vi "SO2 43i Serial Data Recording & DECADEv3.6.vi"() -> ()   [LabVIEW 2014]
uses:
  <vilib>/Instr/_visa.llb/VISA Set IO Buffer Mask.ctl
  <vilib>/Platform/TimedLoop/XDataNode/timing_clust.ctl
  <vilib>/Platform/TimedLoop/XDataNode/nitl_modes.ctl
  <vilib>/Platform/TimedLoop/XDataNode/wakeup.ctl
  C:/Program Files (x86)/National Instruments/LabVIEW 2014/examples/Data Communication/Network Streams/Simple Network Streams/support/Network Stream Command.ctl
  <vilib>/Utility/error.llb/whitespace.ctl
  <vilib>/Instr/_visa.llb/VISA Configure Serial Port (Instr).vi
  <vilib>/Utility/tcp.llb/UDP Multicast Write-Only Open.vi
  <vilib>/platform/TimedLoop/XDataNode/XDataNode.xnode
  <vilib>/Platform/TimedLoop/XDataNode/XDNodeRunTimeDep.lvlib
panel:
  out "Default file name":string
  out "Stop File Write":bool
  out "error out 4":errorcluster
  out "V6":bool
  out "V8":bool
  out "V9":bool
  out "error out 2":errorcluster
  in  "MFC_2 SLPM set value":dbl
  out "Value Read 2":string
  out "status 2":bool
  out "MFC 2":dbl[](array[numeric])
  in  "VISA resource name 3":refnum<visa-resource-name>="ASRL4::INSTR"
  in  "timeout (10sec) 3":u32=3000
  out "error out 3":errorcluster
  in  "MFC_3 SLPM set value":dbl=2.0
  out "Value Read 3":string
  out "status":bool
  out "MFC 3":dbl[](array[numeric])
  in  "VISA resource name 2":refnum<visa-resource-name>="ASRL5::INSTR"
  in  "timeout (10sec) 2":u32=3000
  out "Data Array UDP":string[](array[string])
  out "Slope":dbl=1.0
  out "Offset":dbl
  out "Simulate TWA Conc":dbl
  out "8hr_TWA_limit":i32=490
  out "10mins_STEL_limit":i32=700
  out "Simulate STEL Conc":dbl
  out "Simulate\nconc":bool
  out "q_size 2":i32
  out "8hr_so2_avg 2":dbl=1.0
  out "10min_so2_avg":dbl=1.0
  out "q_size":i32
  in  "Clear Display\nErrors":bool
  in  "dummy2":string="0"
  out "Data Processing":bool
  out "Serial Visa Error":errorcluster
  out "SEPTIC TCP Error Out":errorcluster
  out "TCP packet\nSend to SEPTIC":bool
  out "UDP Time Stamp Offset":i32=1
  out "Data Array TCP":string[](array[string])
  out "UDP packet \nstatus":bool
  out "UDP_Out_Error":errorcluster
  out "FISH TCP Error Out":errorcluster
  out "TCP packet\nSend to FISH":bool
  out "TCP Binary Packet":string
  out "Scan from String Error Counter\nfrom process loop":i32
  out "Read Error Counter\nfrom process loop":i32
  in  "milliseconds to wait":u32=330
  in  "ID":string="µ"
  in  "VISA resource name":refnum<visa-resource-name>="ASRL6::INSTR"
  out "Data In Array":string[](array[string])
  out "UDP_ASCII_Out":string
  out "UDP_Pack_num":u32
  out "Flight Number":string
  in  "dummy1":string="00"
  out "Data String":string
  out "Internal packet":string[](array[string])
  out "RAW DATA":string
  in  "stop":bool
  out "Time taken history":u32(graph)
  out "Max Acq Time diff":u32
  out "Acq Time":u32
  out "Number of Send & Read Error\nfrom Acquire Loop":i32
  out "Command In":string
  # "SO2_conc"
  # "PMT_Volt"
  # "Lamp_Volt"
  # "Lamp_Intensity_Hz"
  # "Internal_Temp_degC"
  # "Reaction_Chamber_Temp_degC"
  # "Reaction_Chamber_Press_mmHg"
  # "Sample_Flow_litre_per_minute"
  # "Flag"
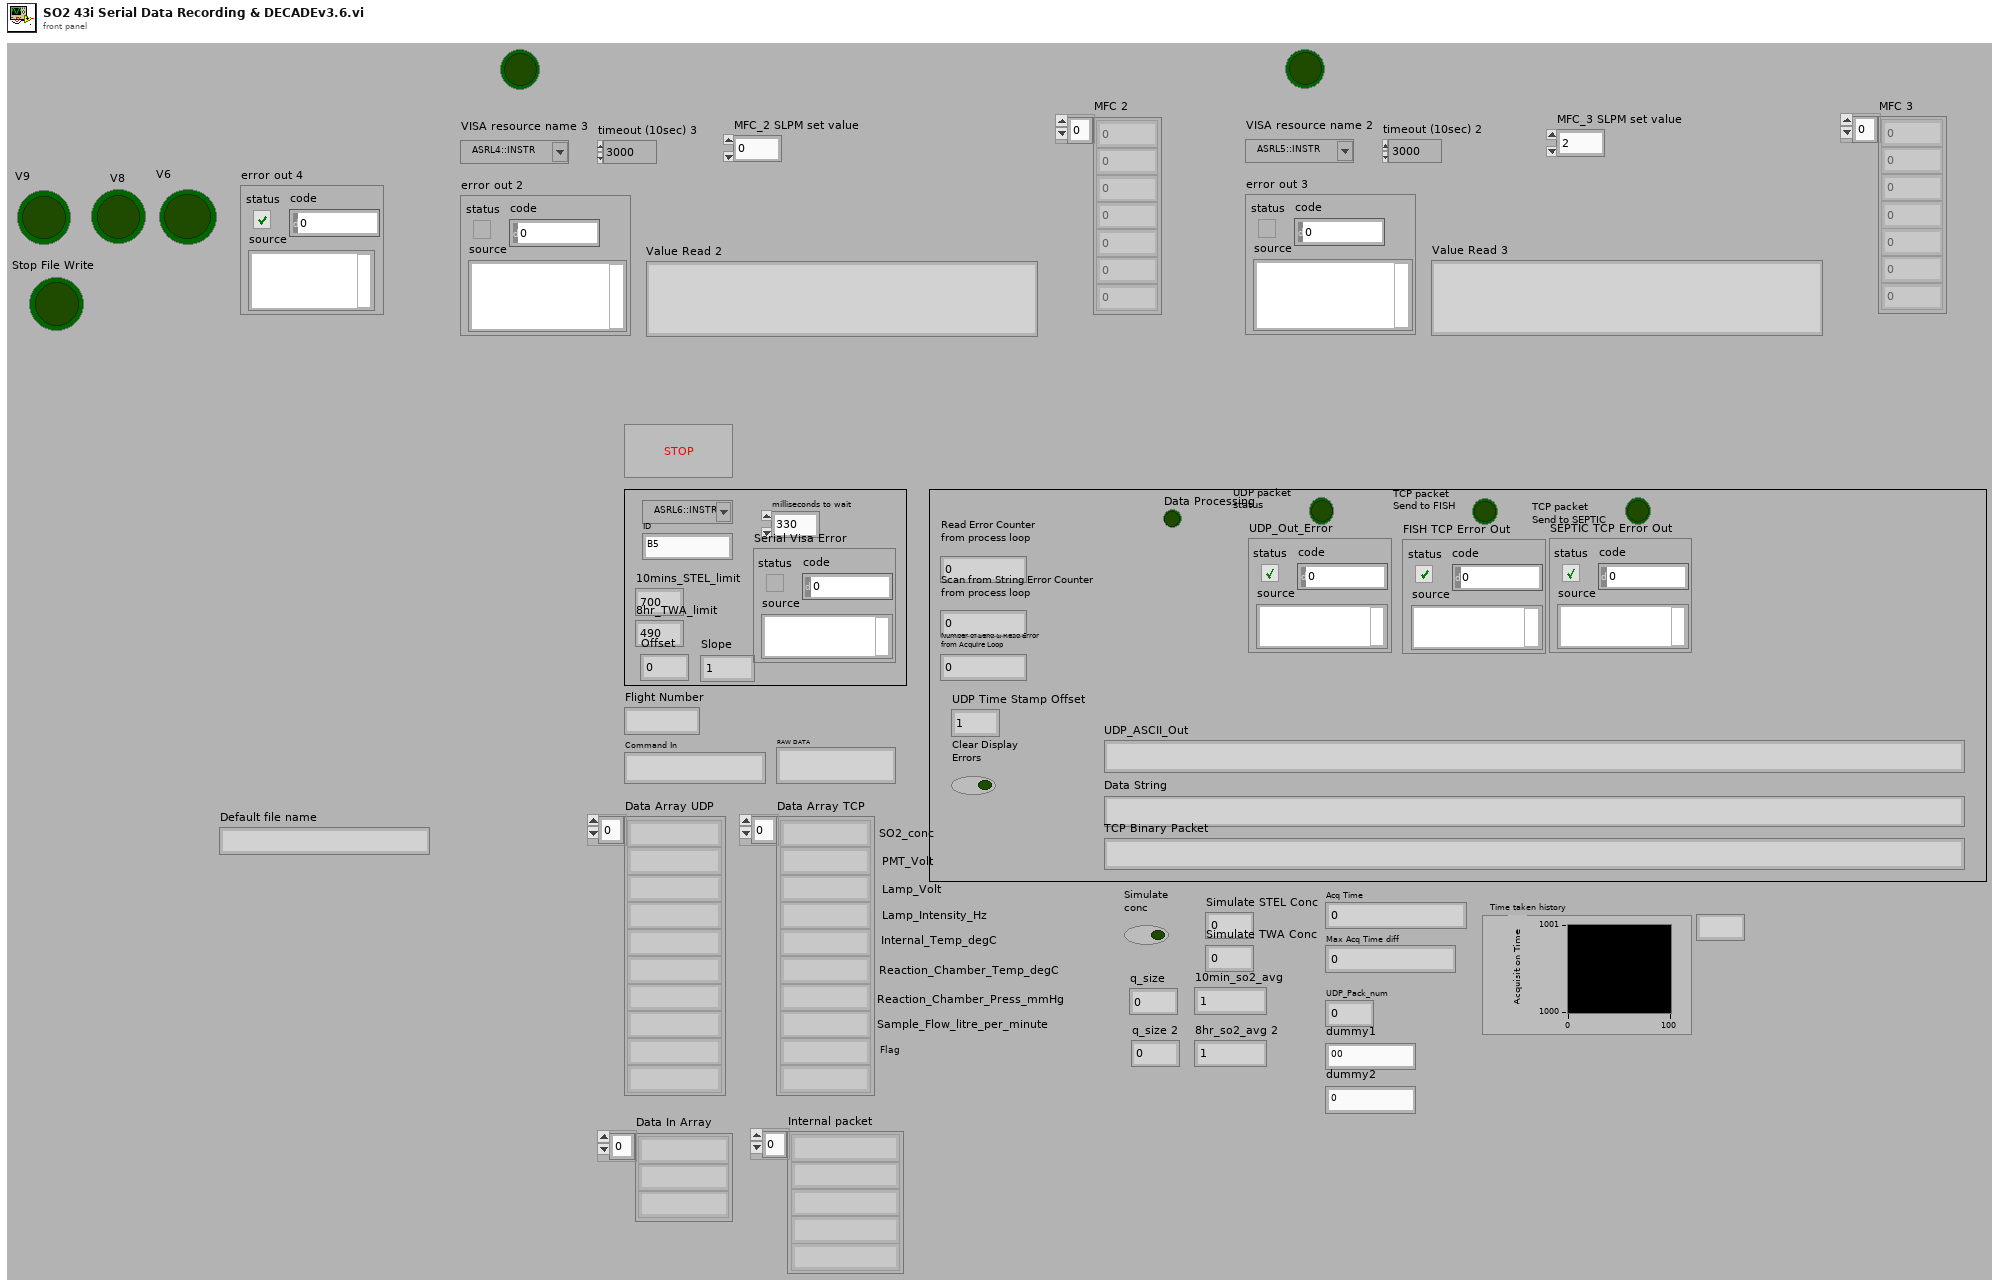
[diagram p1: front panel]
types:
  T1 = typedef "VISA Set IO Buffer Mask.ctl" = u16
  T2 = typedef "Network Stream Command.ctl" = cluster{"Message":string, "Message Data":variant}
  T3 = typedef "XDNodeRunTimeDep.lvlib/timing_clust.ctl" = cluster{"Expected End [f-1]":u64, "Actual End [f-1]":u64, "Finished Late? [f-1]":bool, "Expected End [i-1]":u64, "Actual End [i-1]":u64, "Finished Late? [i-1]":bool, "Expected Start [i]":u64, "Actual Start [i]":u64, "Expected Start [f]":u64, "Actual Start [f]":u64, "Source Name":string, "Structure Name":string, "Period":i64, "Deadline":i64, "Offset":i64, "Start":i64, "Priority":i32, "Timeout":i32, "Mode":T4, "Wakeup Reason":T5, "Error":errorcluster, "Source Type":string, "Secondary Source Type":string, "Global End Time":u64, "Global Start Time":u64, "Frame Duration":u64, "Iteration Duration":u64, "Assigned CPU":i32, "I/O Scan Engine Mode":u32}
  T4 = typedef "XDNodeRunTimeDep.lvlib/nitl_modes.ctl" = enum32{"No Change", "Process missed periods, maintain original phase", "Discard missed periods, maintain original phase", "Process missed periods, ignore original phase", "Discard missed periods, ignore original phase"}
  T5 = typedef "XDNodeRunTimeDep.lvlib/wakeup.ctl" = enum32{"Normal", "Aborted", "Asynchronous wakeup", "Timing source error", "Timed loop error", "Timeout"}
  T6 = enum16{"open", "replace", "create", "open or create", "replace or create", "replace or create with confirmation"}
  T7 = typedef "whitespace.ctl" = u16
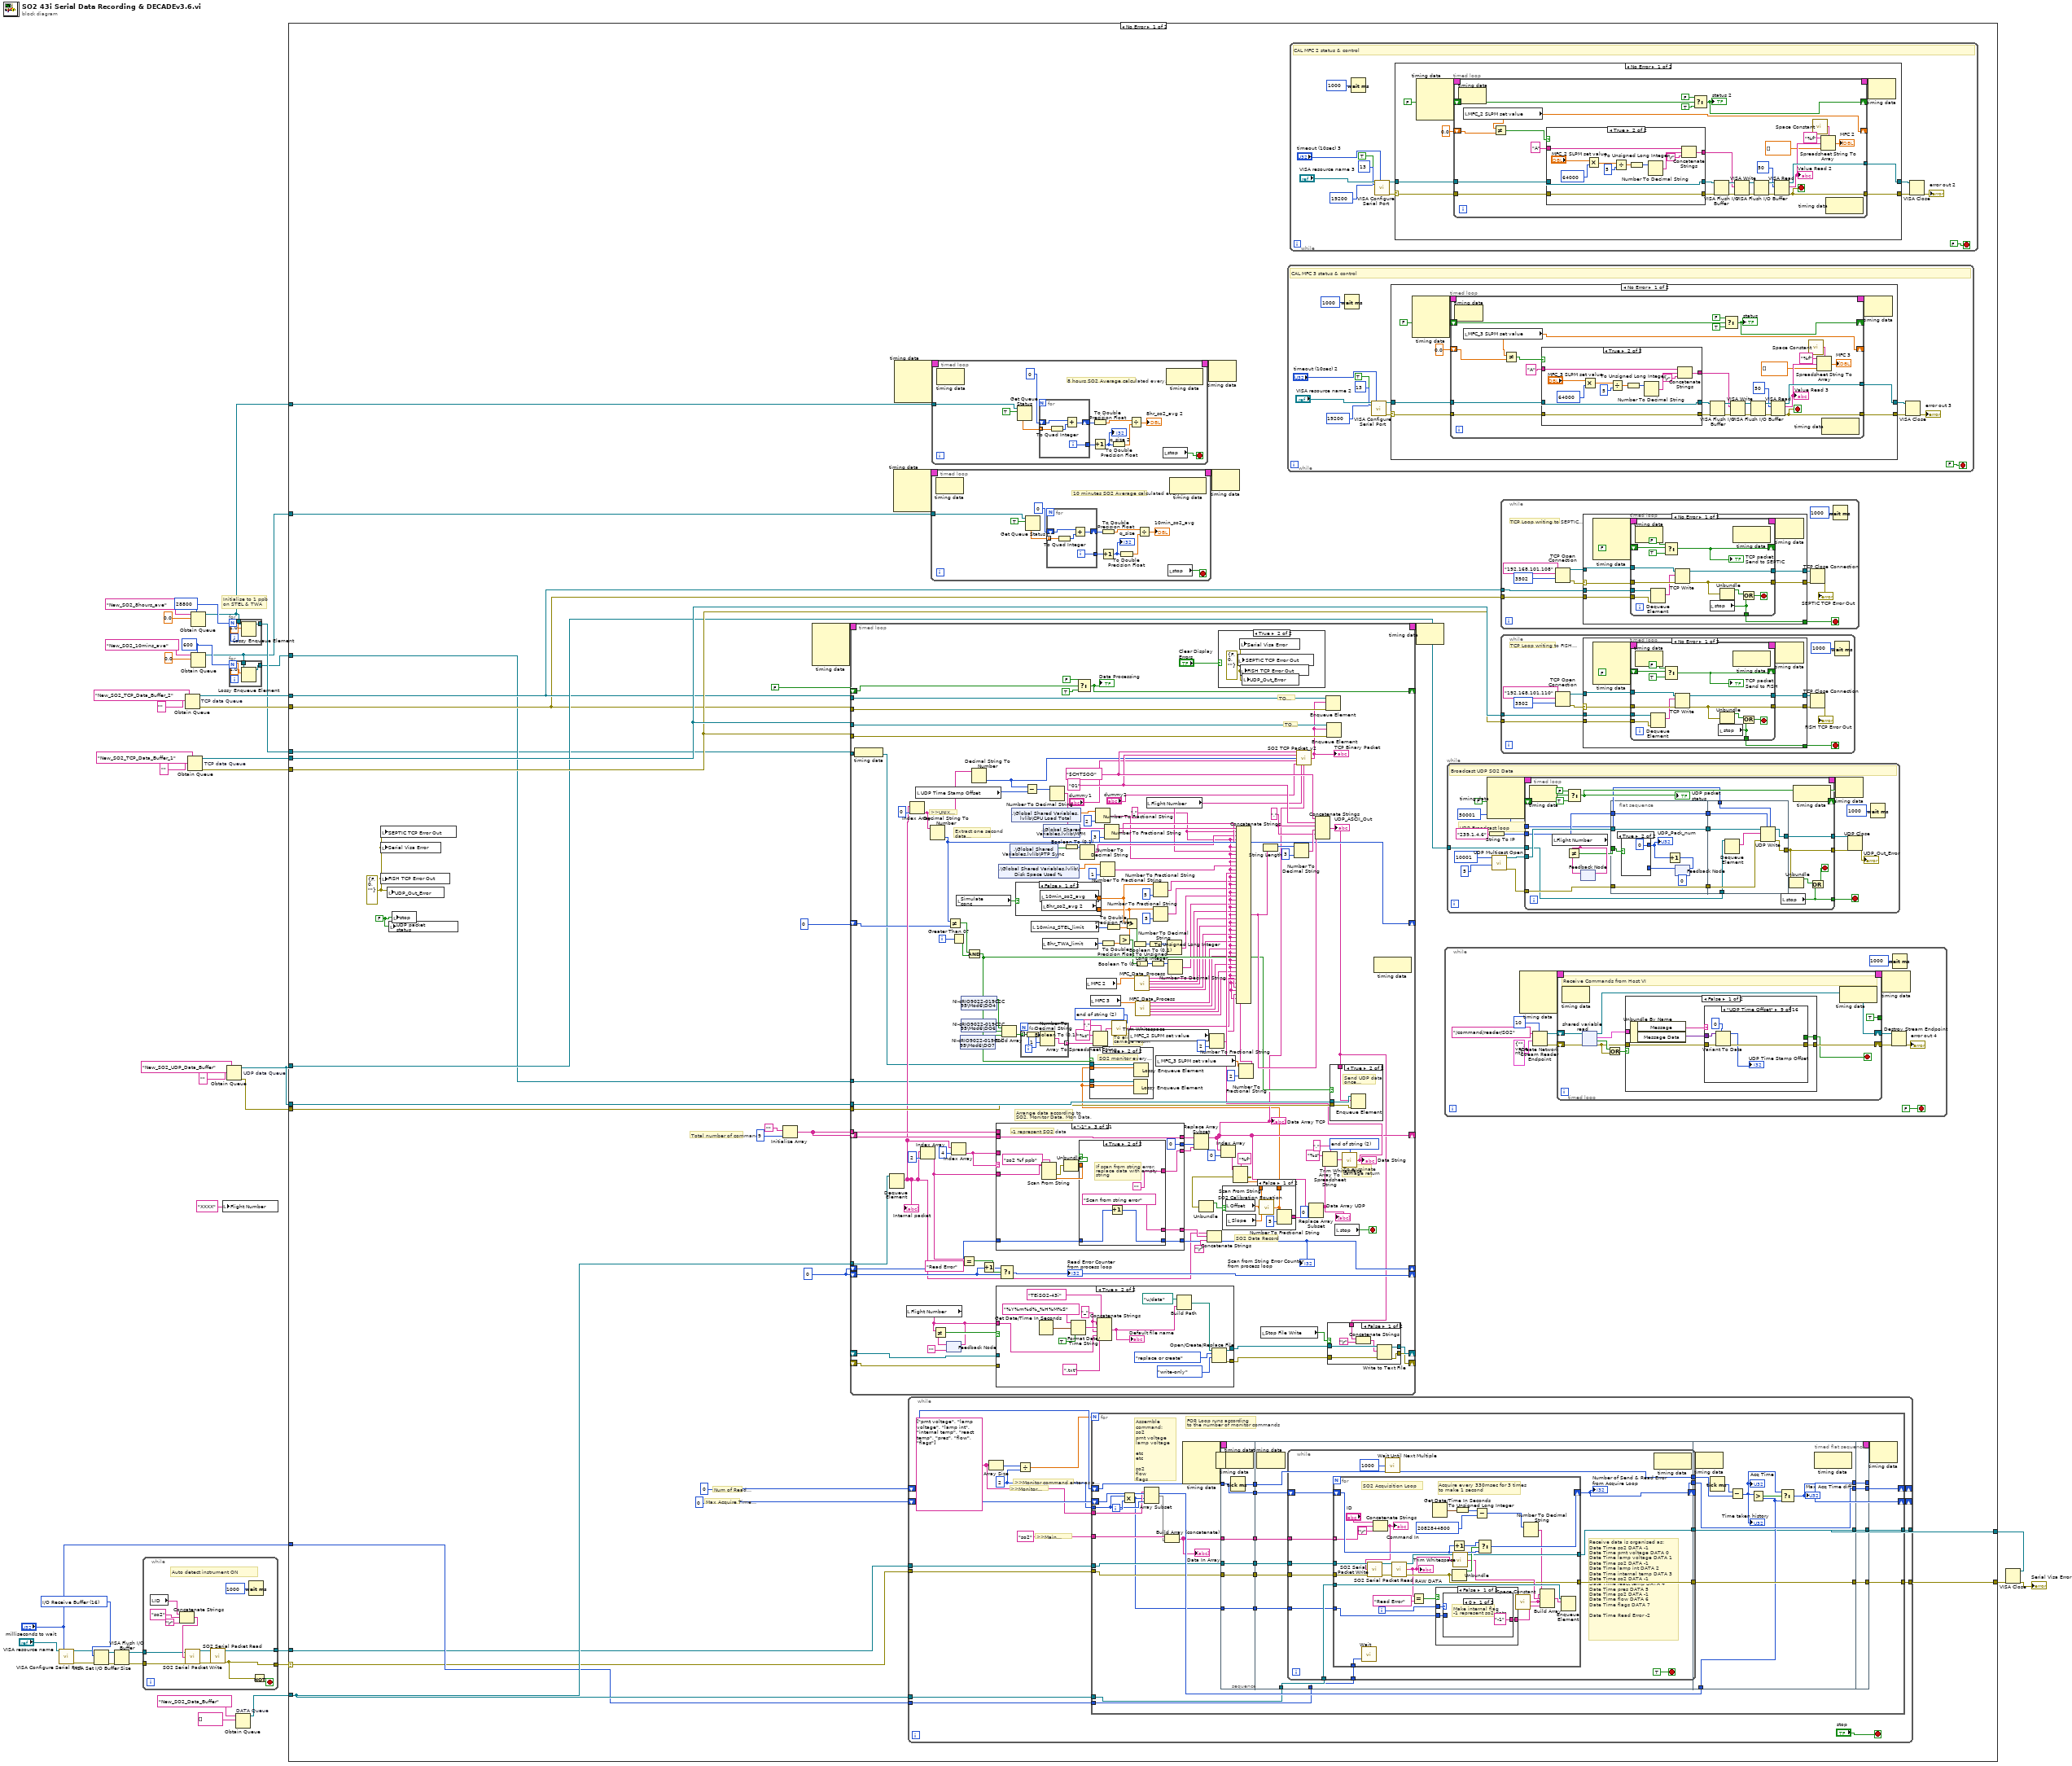
[diagram p0: block diagram]
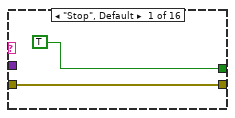
[diagram p2: hidden frame]
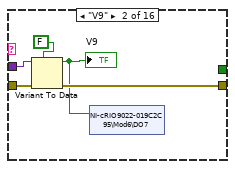
[diagram p3: hidden frame]
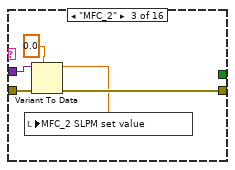
[diagram p4: hidden frame]
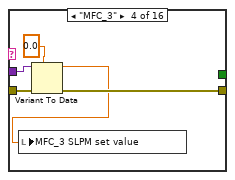
[diagram p5: hidden frame]
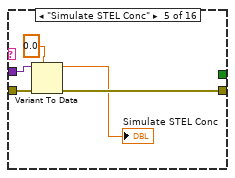
[diagram p6: hidden frame]
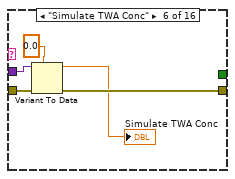
[diagram p7: hidden frame]
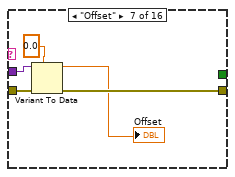
[diagram p8: hidden frame]
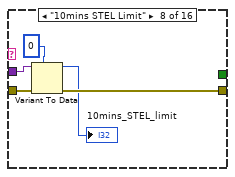
[diagram p9: hidden frame]
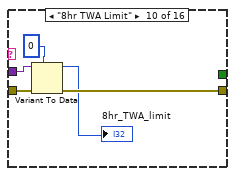
[diagram p10: hidden frame]
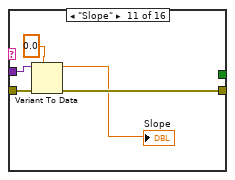
[diagram p11: hidden frame]
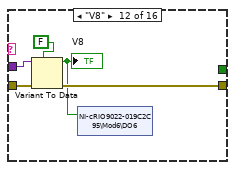
[diagram p12: hidden frame]
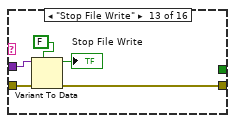
[diagram p13: hidden frame]
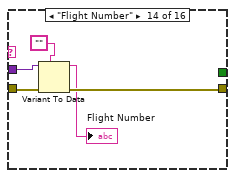
[diagram p14: hidden frame]
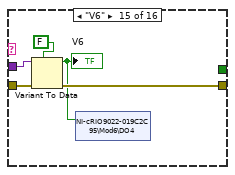
[diagram p15: hidden frame]
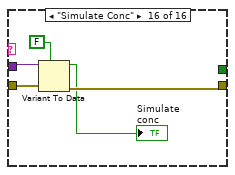
[diagram p16: hidden frame]
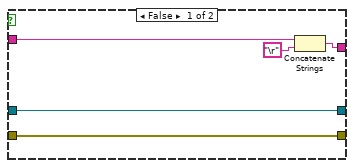
[diagram p18: hidden frame]
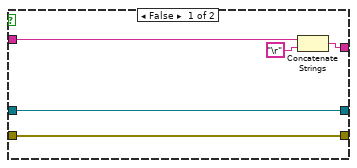
[diagram p20: hidden frame]
diagram:
  w9 = T1 16 items=["I/O Receive Buffer"=16, "I/O Transmit Buffer"=32, "I/O Receive and Transmit Buffer"=48] ("Mask")
  w16 = 28800 ("max queue size (-1, unlimited)")
  w13 = 600 ("max queue size (-1, unlimited)")
  # "Initialise to 1 ppb\non STEL & TWA"
  n1 = call-poly "VISA Configure Serial Port"("VISA resource name"="VISA resource name", "timeout (10sec)"="milliseconds to wait") -> ("VISA resource name out"=w8:refnum<visa-resource-name>, "error out"=w7:errorcluster)  [unwired: 12 in]
  n2 = VISA Set I/O Buffer Size(VISA resource name=w8, mask (16)=w9, error in (no error)=w7) -> (VISA resource name out=w2:refnum<visa-resource-name>, error out=w10:errorcluster)  [unwired: 1 in]
  n3 = VISA Flush I/O Buffer(VISA resource name=w2, error in (no error)=w10) -> (VISA resource name out=w6:refnum<visa-resource-name>, error out=w5:errorcluster)  [unwired: 1 in]
  n4 = while {
    tunnel: w6 -> [w45]
    tunnel: w5 -> [w44]
    tunnel: [w43] -> w4
    tunnel: [w42] -> w3
    stop <- w41 stop-if-true
    # "Auto detect instrument ON"
    n5 = local read "ID"() -> (w46:string)
    n6 = Concatenate Strings(w46, "so2" ("string"), "\r") -> (w49:string)
    n7 = call "SO2 Serial Packet Write.vi"("VISA resource name In"=w45, "Data in"=w49, "error in (no error)"=w44) -> ("VISA resource name Out"=w51:refnum<visa-resource-name>, "error out"=w50:errorcluster)  [unwired: 11 in]
    n8 = call "SO2 Serial Packet Read.vi"("VISA resource In"=w51, "error in"=w50) -> ("VISA resource Out"=w42:refnum<visa-resource-name>, "error out"=w43:errorcluster)  [unwired: 11 in, 1 out]
    n9 = Wait (ms)(milliseconds to wait=u32 1000) -> ()  [unwired: 1 out]
    n10 = Not(x=w43) -> (.not. x?=w41:bool)
  }
  n11 = Obtain Queue "TCP data Queue"(name (unnamed)="New_SO2_TCP_Data_Buffer_2", element data type="") -> (queue out=w23:refnum<queue>, error out=w22:errorcluster)  [unwired: 3 in, 1 out]
  n12 = Obtain Queue "TCP data Queue"(name (unnamed)="New_SO2_TCP_Data_Buffer_1", element data type="") -> (queue out=w31:refnum<queue>, error out=w30:errorcluster)  [unwired: 3 in, 1 out]
  n13 = Obtain Queue(max queue size (-1, unlimited)=w16, name (unnamed)="New_SO2_8hours_ave", element data type=0.0 ("index")) -> (queue out=w15:refnum<queue>)  [unwired: 2 in, 2 out]
  n14 = Obtain Queue(max queue size (-1, unlimited)=w13, name (unnamed)="New_SO2_10mins_ave", element data type=0.0 ("index")) -> (queue out=w12:refnum<queue>)  [unwired: 2 in, 2 out]
  n15 = local write "Flight Number"("XXXX" ("Flight Number")) -> ()
  n16 = Obtain Queue "UDP data Queue"(name (unnamed)="New_SO2_UDP_Data_Buffer", element data type="") -> (queue out=w26:refnum<queue>, error out=w27:errorcluster)  [unwired: 3 in, 1 out]
  n17 = for {
    N: w16 -> [_]
    tunnel: w15 -> [w55]
    tunnel: [w54] -> w14
    n18 = Lossy Enqueue Element(queue=w55, element=1.0) -> (queue out=w54:refnum<queue>)  [unwired: 1 in, 3 out]
  }
  n19 = for {
    N: w13 -> [_]
    tunnel: [w58] -> w11
    tunnel: w12 -> [w56]
    n20 = Lossy Enqueue Element(queue=w56, element=1.0) -> (queue out=w58:refnum<queue>)  [unwired: 1 in, 3 out]
  }
  n21 = Obtain Queue "DATA Queue"(name (unnamed)="New_SO2_Data_Buffer", element data type=string[] []) -> (queue out=w38:refnum<queue>)  [unwired: 3 in, 2 out]
  n22 = case shown="No Error" w4 {
    selector: w4 -> [w59 w1070]
    tunnel: [w91 w1070] -> w35
    tunnel: [w90 w1069] -> w36
    tunnel: w38 -> [w87 _]
    tunnel: w3 -> [w60 w1069]
    tunnel: w31 -> [w79 _]
    tunnel: w30 -> [w78 _]
    tunnel: w26 -> [w77 _]
    tunnel: w27 -> [w76 _]
    tunnel: w26 -> [w75 _]
    tunnel: w23 -> [w73 _]
    tunnel: w22 -> [w72 _]
    tunnel: "milliseconds to wait" -> [w71 _]
    tunnel: w12 -> [w68 _]
    tunnel: w15 -> [w67 _]
    tunnel: w11 -> [w66 _]
    tunnel: w14 -> [w65 _]
    frame No Error {
      w69 = errorcluster {"status"=FALSE, "code"=0, "source"=""} ("UDP Error Out")
      w81 = 0
      w80 = FALSE ("stop")
      # "Max Acquire Time Diff"
      # "Num of Read Error"
      # "Total number of commands"
      n23 = local write "SEPTIC TCP Error Out"(w69) -> ()
      n24 = local write "Serial Visa Error"(w69) -> ()
      n25 = local write "FISH TCP Error Out"(w69) -> ()
      n26 = local write "UDP_Out_Error"(w69) -> ()
      n27 = local write "UDP packet \nstatus"(w80) -> ()
      n28 = local write "stop"(w80) -> ()
      n29 = Initialize Array("", 9) -> (w82:string[])
      n30 = node-c288() -> (w89:T3)  [unwired: 4 in]
      n31 = timed-loop {
        timing: w89 -> [_]
        timing-out: [_] -> w88
        tunnel: w87 -> [w812]
        shift-right: [w731] -> _
        shift-left: w82 -> [w802]
        shift-right: [w793] -> _
        shift-left: w81 -> [w790]
        tunnel: w82 -> [w792]
        shift-right: [w788] -> _
        shift-left: w81 -> [w789]
        tunnel: w79 -> [w783]
        tunnel: w78 -> [w782]
        tunnel: w77 -> [w781]
        tunnel: w76 -> [w780]
        shift-right: [w772] -> _
        shift-left: 0 -> [w775]
        tunnel: w73 -> [w771]
        tunnel: w72 -> [w770]
        shift-right: [w762] -> _
        shift-left: FALSE -> [w765]
        tunnel: w66 -> [w756]
        tunnel: w65 -> [w755]
        shift-right: [w702] -> _
        shift-left: _ -> [w704]
        shift-right: [w701] -> _
        shift-left: _ -> [w703]
        i -> [w773]
        stop <- w810 stop-if-true
        w672 = T7 2 items=["both", "start of string", "end of string"] ("location (both)")
        w798 = T7 2 items=["both", "start of string", "end of string"] ("location (both)")
        w668 = ","
        w785 = "01"
        w804 = ","
        w786 = "$CHTSOO"
        # "To eliminate\ncarriage return"
        # "TO SEPTIC"
        # "TO FISH"
        # "Extract one second data\nfor UDP sending"
        # "Arrange data according to\nSO2, Monitor Data, Mon Data,"
        # "To eliminate\ncarriage return"
        # ">>UNIX TIME>>"
        # "SO2 Data Record"
        n32 = node-c288() -> ()  [unwired: 1 in]
        n33 = Dequeue Element(queue=w812) -> (element=w778:string[])  [unwired: 2 in, 3 out]
        "Internal packet" <- w778
        n34 = local read "Flight Number"() -> (w705:string)
        n35 = Index Array(array=w778, index=0) -> (element=w777:string)
        n36 = local read "UDP Time Stamp Offset"() -> (w671:i32)
        n37 = Index Array(array=w778, index=2) -> (element=w796:string)
        n38 = Decimal String To Number(string=w777) -> (number=w772:i32)  [unwired: 2 in, 1 out]
        n39 = feedback #1("" ("Flight Number")) -> (w710:string)
        n40 = Not Equal?(x=w705, y=w710) -> (x != y?=w708:bool)
        n41 = feedback-in #1(w705) -> ()
        n42 = Not Equal?(x=w772, y=w775) -> (x != y?=w774:bool)
        n43 = Index Array(array=w778, index=4) -> (element=w761:string)
        n44 = Greater Than 0?(x=w773) -> (x > 0?=w776:bool)
        n45 = local read "Simulate\nconc"() -> (w713:bool)
        n46 = shared-variable "NI-cRIO9022-019C2C95\\Mod6\\DO7"() -> (w685:bool)  [unwired: 1 in, 1 out]
        n47 = shared-variable "NI-cRIO9022-019C2C95\\Mod6\\DO6"() -> (w686:bool)  [unwired: 1 in, 1 out]
        n48 = shared-variable "NI-cRIO9022-019C2C95\\Mod6\\DO4"() -> (w687:bool)  [unwired: 1 in, 1 out]
        n49 = Equal?(x=w796, y="Read Error") -> (x = y?=w794:bool)
        n50 = Compound Arithmetic op=AND(w774, w776) -> (w757:bool)
        n51 = Decimal String To Number(string=w777) -> (number=w767:i32)  [unwired: 2 in, 1 out]
        n52 = Increment(x=w790) -> (x+1=w791:i32)
        n53 = case shown="True" w708 {
          tunnel: [w818 w821] -> w707
          tunnel: [w817 w820] -> w706
          tunnel: w704 -> [w818 _]
          tunnel: w703 -> [w817 _]
          tunnel: w705 -> [_ w819]
          frame False {
          }
          frame True {
            w828 = "_" ("string")
            n54 = Get Date/Time In Seconds() -> (seconds since 1Jan1904=w829:timestamp)
            n55 = Format Date/Time String(time format string (%c)="%Y%m%d%_%H%M%S", seconds (now)=w829, UTC format=TRUE) -> (date/time string=w832:string)
            n56 = Concatenate Strings("TEiSO2-43i" ("string"), w828, w832, w828, w819, ".txt" ("string")) -> (w826:string)
            "Default file name" <- w826
            n57 = Build Path(base path=path "u:/data", name or relative path=w826) -> (appended path=w822:path)
            n58 = Open/Create/Replace File(file path (use dialog)=w822, operation (0:open)=T6."replace or create", access (0:read/write)=enum16{"read/write", "read-only", "write-only"}."write-only") -> (refnum out=w821:refnum<file>, error out=w820:errorcluster)  [unwired: 3 in, 1 out]
          }
        }
        n59 = case shown="\"-1\"" w761 {
          tunnel: w761 -> [w868 _ _ w904 w925 w946 w968 w990 w1012 w1034 w1056]
          tunnel: w802 -> [w869 _ w883 w905 w926 w947 w969 w991 w1013 w1035 w1057]
          tunnel: w796 -> [_ _ w880 w900 w921 w943 w965 w987 w1009 w1031 w1053]
          tunnel: [w869 w872 w883 w905 w926 w947 w969 w991 w1013 w1035 w1057] -> w738
          tunnel: [w866 _ 0 ("index") w902 w923 w944 w966 w988 w1010 w1032 w1054] -> w737
          tunnel: [_ _ w879 w899 w920 w942 w964 w986 w1008 w1030 w1048] -> w801
          tunnel: w792 -> [_ w872 _ _ _ _ _ _ _ _ _]
          tunnel: w789 -> [w864 w871 w876 w896 w917 w937 w960 w981 w1004 w1025 w1047]
          tunnel: [w864 w871 w875 w895 w916 w936 w959 w980 w1003 w1024 w1046] -> w788
          tunnel: ["Internal False Flag Detected" "" w874 w894 w915 w935 w958 w979 w1002 w1023 w1045] -> w787
          frame "False", Default {
            n60 = Decimal String To Number(string=w868) -> (number=w865:i32)  [unwired: 2 in, 1 out]
            n61 = Add(x=w865, y=1) -> (x+y=w866:i32)
          }
          frame "-2" {
            # "Read Error Detected\nMake all data as a space"
          }
          frame "-1" {
            # "-1 represent SO2 data"
            n62 = Scan From String(format string="so2 %f ppb", input string=w880) -> (error out=w878:errorcluster, output 1=w873:dbl)  [unwired: 3 in, 2 out]
            n63 = Unbundle(w878) -> ("status"=w877:bool)  [unwired: 2 out]
            n64 = case shown="True" w877 {
              tunnel: w873 -> [w884 _]
              tunnel: [w888 ""] -> w879
              tunnel: w876 -> [w887 w892]
              tunnel: [w887 w891] -> w875
              tunnel: ["" "Scan from string error"] -> w874
              frame False {
                # "Extract the concentration\nvalue & fixed format"
                n65 = Number To Fractional String(number=w884, precision (6)=i16 5) -> (F-format string=w888:string)  [unwired: 2 in]
              }
              frame True {
                # "If scan from string error,\nreplace data with empty\nstring"
                n66 = Increment(x=w892) -> (x+1=w891:i32)
              }
            }
          }
          frame "0" {
            # "0 represents pmt voltage -0510 volts"
            n67 = Scan From String(format string="pmt voltage %d", input string=w900) -> (error out=w898:errorcluster, output 1=w893:i32)  [unwired: 3 in, 2 out]
            n68 = Decimal String To Number(string=w904) -> (number=w903:i32)  [unwired: 2 in, 1 out]
            n69 = Unbundle(w898) -> ("status"=w897:bool)  [unwired: 2 out]
            n70 = case shown="False" w897 {
              tunnel: w893 -> [w909 _]
              tunnel: [w906 w910] -> w899
              tunnel: w896 -> [w908 w913]
              tunnel: [w908 w912] -> w895
              tunnel: ["" "Scan from string error"] -> w894
              tunnel: [w906 w910] -> _
              frame False {
                # "Extract the actual value\n& fixed format"
                n71 = Number To Decimal String(number=w909) -> (decimal integer string=w906:string)  [unwired: 1 in]
              }
              frame True {
                w910 = ""
                # "If scan from string error,\nreplace data with empty\nstring"
                n72 = Increment(x=w913) -> (x+1=w912:i32)
              }
            }
            n73 = Increment(x=w903) -> (x+1=w902:i32)
          }
          frame "1" {
            # "1 represents lamp voltage; lamp voltage 810 volts"
            n74 = Scan From String(format string="lamp voltage %d", input string=w921) -> (error out=w919:errorcluster, output 1=w914:i32)  [unwired: 3 in, 2 out]
            n75 = Decimal String To Number(string=w925) -> (number=w924:i32)  [unwired: 2 in, 1 out]
            n76 = Unbundle(w919) -> ("status"=w918:bool)  [unwired: 2 out]
            n77 = case shown="True" w918 {
              tunnel: w914 -> [w930 _]
              tunnel: [w927 w931] -> w920
              tunnel: w917 -> [w929 w934]
              tunnel: [w929 w933] -> w916
              tunnel: ["" "Scan from string error"] -> w915
              tunnel: [w927 w931] -> _
              frame False {
                # "Extract the actual value\n& fixed format"
                n78 = Number To Decimal String(number=w930) -> (decimal integer string=w927:string)  [unwired: 1 in]
              }
              frame True {
                w931 = ""
                # "If scan from string error,\nreplace data with empty\nstring"
                n79 = Increment(x=w934) -> (x+1=w933:i32)
              }
            }
            n80 = Increment(x=w924) -> (x+1=w923:i32)
          }
          frame "2" {
            # "2 represents lamp intensity; lamp int 35867 Hz"
            n81 = Scan From String(format string="lamp int %d", input string=w943) -> (error out=w939:errorcluster, output 1=w940:i32)  [unwired: 3 in, 2 out]
            n82 = Decimal String To Number(string=w946) -> (number=w945:i32)  [unwired: 2 in, 1 out]
            n83 = Unbundle(w939) -> ("status"=w938:bool)  [unwired: 2 out]
            n84 = case shown="True" w938 {
              tunnel: [w948 w953] -> w942
              tunnel: w940 -> [w952 _]
              tunnel: w937 -> [w951 w956]
              tunnel: [w951 w955] -> w936
              tunnel: ["" "Scan from string error"] -> w935
              tunnel: [w948 w953] -> _
              frame False {
                # "Extract the actual value\n& fixed format"
                n85 = Number To Fractional String(number=w952, precision (6)=i16 0) -> (F-format string=w948:string)  [unwired: 2 in]
              }
              frame True {
                w953 = ""
                # "If scan from string error,\nreplace data with empty\nstring"
                n86 = Increment(x=w956) -> (x+1=w955:i32)
              }
            }
            n87 = Increment(x=w945) -> (x+1=w944:i32)
          }
          frame "3" {
            # "3 represents internal temp; internal temp 027.2 deg C, actual 027.2"
            n88 = Scan From String(format string="%[^,], %s %f", input string=w965) -> (error out=w962:errorcluster, output 3=w957:dbl)  [unwired: 7 in, 2 out]
            n89 = Decimal String To Number(string=w968) -> (number=w967:i32)  [unwired: 2 in, 1 out]
            n90 = Unbundle(w962) -> ("status"=w961:bool)  [unwired: 2 out]
            n91 = case shown="True" w961 {
              tunnel: [w970 w975] -> w964
              tunnel: w957 -> [w974 _]
              tunnel: w960 -> [w973 w978]
              tunnel: [w973 w977] -> w959
              tunnel: ["" "Scan from string error"] -> w958
              tunnel: [w970 w975] -> _
              frame False {
                # "Extract the actual value\n& fixed format"
                n92 = Number To Fractional String(number=w974, precision (6)=i16 1) -> (F-format string=w970:string)  [unwired: 2 in]
              }
              frame True {
                w975 = ""
                # "If scan from string error,\nreplace data with empty\nstring"
                n93 = Increment(x=w978) -> (x+1=w977:i32)
              }
            }
            n94 = Increment(x=w967) -> (x+1=w966:i32)
          }
          frame "4" {
            # "4 represents react temp; react temp 045.2 deg C"
            n95 = Scan From String(format string="react temp %f deg C", input string=w987) -> (error out=w983:errorcluster, output 1=w984:dbl)  [unwired: 3 in, 2 out]
            n96 = Decimal String To Number(string=w990) -> (number=w989:i32)  [unwired: 2 in, 1 out]
            n97 = Unbundle(w983) -> ("status"=w982:bool)  [unwired: 2 out]
            n98 = case shown="False" w982 {
              tunnel: [w992 w997] -> w986
              tunnel: w984 -> [w996 _]
              tunnel: w981 -> [w995 w1000]
              tunnel: [w995 w999] -> w980
              tunnel: ["" "Scan from string error"] -> w979
              tunnel: [w992 w997] -> _
              frame False {
                # "Extract the actual value\n& fixed format"
                n99 = Number To Fractional String(number=w996, precision (6)=i16 1) -> (F-format string=w992:string)  [unwired: 2 in]
              }
              frame True {
                w997 = ""
                # "If scan from string error,\nreplace data with empty\nstring"
                n100 = Increment(x=w1000) -> (x+1=w999:i32)
              }
            }
            n101 = Increment(x=w989) -> (x+1=w988:i32)
          }
          frame "5" {
            # "5 represents chamber pressure; pres 760.0 mm Hg, actual 753.4"
            n102 = Scan From String(format string="%[^,], %s %f", input string=w1009) -> (error out=w1006:errorcluster, output 3=w1001:dbl)  [unwired: 7 in, 2 out]
            n103 = Decimal String To Number(string=w1012) -> (number=w1011:i32)  [unwired: 2 in, 1 out]
            n104 = Unbundle(w1006) -> ("status"=w1005:bool)  [unwired: 2 out]
            n105 = case shown="False" w1005 {
              tunnel: [w1014 w1019] -> w1008
              tunnel: w1001 -> [w1018 _]
              tunnel: w1004 -> [w1017 w1022]
              tunnel: [w1017 w1021] -> w1003
              tunnel: ["" "Scan from string error"] -> w1002
              tunnel: [w1014 w1019] -> _
              frame False {
                # "Extract the actual value\n& fixed format"
                n106 = Number To Fractional String(number=w1018, precision (6)=i16 1) -> (F-format string=w1014:string)  [unwired: 2 in]
              }
              frame True {
                w1019 = ""
                # "If scan from string error,\nreplace data with empty\nstring"
                n107 = Increment(x=w1022) -> (x+1=w1021:i32)
              }
            }
            n108 = Increment(x=w1011) -> (x+1=w1010:i32)
          }
          frame "6" {
            # "6 represents flow data; flow 0.503 l/m"
            n109 = Scan From String(format string="flow %f l/m", input string=w1031) -> (error out=w1027:errorcluster, output 1=w1028:dbl)  [unwired: 3 in, 2 out]
            n110 = Decimal String To Number(string=w1034) -> (number=w1033:i32)  [unwired: 2 in, 1 out]
            n111 = Unbundle(w1027) -> ("status"=w1026:bool)  [unwired: 2 out]
            n112 = case shown="True" w1026 {
              tunnel: [w1040 ""] -> w1030
              tunnel: w1028 -> [w1039 _]
              tunnel: w1025 -> [w1038 w1043]
              tunnel: [w1038 w1042] -> w1024
              tunnel: ["" "Scan from string error"] -> w1023
              frame False {
                # "Extract the actual value\n& fixed format"
                n113 = Number To Fractional String(number=w1039, precision (6)=i16 3) -> (F-format string=w1040:string)  [unwired: 2 in]
              }
              frame True {
                # "If scan from string error,\nreplace data with empty\nstring"
                n114 = Increment(x=w1043) -> (x+1=w1042:i32)
              }
            }
            n115 = Increment(x=w1033) -> (x+1=w1032:i32)
          }
          frame "7" {
            # "7 represents flags data; flags 1c100000"
            n116 = Scan From String(format string="flags %s", input string=w1053) -> (error out=w1051:errorcluster, output 1=w1049:string)  [unwired: 3 in, 2 out]
            n117 = Decimal String To Number(string=w1056) -> (number=w1055:i32)  [unwired: 2 in, 1 out]
            n118 = Unbundle(w1051) -> ("status"=w1050:bool)  [unwired: 2 out]
            n119 = case shown="False" w1050 {
              tunnel: w1049 -> [w1060 _]
              tunnel: [w1060 ""] -> w1048
              tunnel: w1047 -> [w1059 w1063]
              tunnel: [w1059 w1062] -> w1046
              tunnel: ["" "Scan from string error"] -> w1045
              frame False {
                # "Extract the actual value\n& fixed format"
              }
              frame True {
                # "If scan from string error,\nreplace data with empty\nstring"
                n120 = Increment(x=w1063) -> (x+1=w1062:i32)
              }
            }
            n121 = Increment(x=w1055) -> (x+1=w1054:i32)
          }
        }
        "Scan from String Error Counter\nfrom process loop" <- w788
        n122 = shared-variable ".\\Global Shared Variables.lvlib\\Disk Space Used %"() -> (w675:dbl)  [unwired: 1 in, 1 out]
        n123 = Select(t=w791, s=w794, f=w790) -> (s? t:f=w793:i32)
        "Read Error Counter\nfrom process loop" <- w793
        n124 = Build Array(w687, w686, w685) -> (w691:bool[])
        n125 = shared-variable ".\\Global Shared Variables.lvlib\\PTP Sync"() -> (w693:bool)  [unwired: 1 in, 1 out]
        n126 = shared-variable ".\\Global Shared Variables.lvlib\\CPU Load Total"() -> (w698:dbl)  [unwired: 1 in, 1 out]
        n127 = case shown="False" w713 {
          tunnel: [w852 w853] -> w751
          tunnel: [w851 w854] -> w749
          frame False {
            n128 = local read "10min_so2_avg"() -> (w852:dbl)
            n129 = local read "8hr_so2_avg 2"() -> (w851:dbl)
          }
          frame True {
            n130 = local read "Simulate STEL Conc"() -> (w853:dbl)
            n131 = local read "Simulate TWA Conc"() -> (w854:dbl)
          }
        }
        n132 = for {
          tunnel: w691 -> [w815] mode=indexing
          tunnel: [w814] -> w688 mode=indexing
          n133 = Boolean To (0,1)(Boolean=w815) -> (0, 1=w816:i16)
          n134 = Number To Decimal String(number=w816, width (-)=i16 1) -> (decimal integer string=w814:string)
        }
        n135 = Subtract(x=w767, y=w671) -> (x-y=w768:i32)
        n136 = local read "10mins_STEL_limit"() -> (w711:i32)
        n137 = local read "8hr_TWA_limit"() -> (w712:i32)
        n138 = shared-variable ".\\Global Shared Variables.lvlib\\MFM"() -> (w695:dbl)  [unwired: 1 in, 1 out]
        n139 = Number To Decimal String(number=w768) -> (decimal integer string=w766:string)  [unwired: 1 in]
        n140 = Boolean To (0,1)(Boolean=w693) -> (0, 1=w692:i16)
        n141 = Select(t=FALSE, s=w765, f=TRUE) -> (s? t:f=w762:bool)
        "Data Processing" <- w762
        n142 = Number To Decimal String(number=w692) -> (decimal integer string=w678:string)  [unwired: 1 in]
        n143 = local read "MFC 2"() -> (w725:dbl[])
        n144 = local read "MFC 3"() -> (w724:dbl[])
        n145 = Array To Spreadsheet String(delimiter (Tab)=",", array=w688, 3:"%s" ("format string")) -> (spreadsheet string=w673:string)
        n146 = Number To Fractional String(number=w698, precision (6)=i16 2) -> (F-format string=w670:string)  [unwired: 2 in]
        n147 = Number To Fractional String(number=w675, precision (6)=i16 1) -> (F-format string=w669:string)  [unwired: 2 in]
        n148 = To Double Precision Float(number=w712) -> (double precision float=w752:dbl)
        n149 = Number To Fractional String(number=w695, precision (6)=i16 3) -> (F-format string=w694:string)  [unwired: 2 in]
        n150 = To Double Precision Float(number=w711) -> (double precision float=w753:dbl)
        n151 = call <vilib>:"Trim Whitespace.vi"("string"=w673, "location (both)"=w672) -> ("trimmed string"=w674:string)
        n152 = Greater?(x=w749, y=w752) -> (0:w742:bool)
        n153 = Greater?(x=w751, y=w753) -> (0:w744:bool)
        n154 = local read "MFC_2 SLPM set value"() -> (w682:dbl)
        n155 = Boolean To (0,1)(Boolean=w744) -> (0, 1=w746:i16)
        n156 = Boolean To (0,1)(Boolean=w742) -> (0, 1=w745:i16)
        n157 = call "MFC_Data_Process.vi"("MFC"=w725) -> ("MFC Absolute Pressure"=w723:string, "MFC Temperature"=w722:string, "MFC Volumetric Flow"=w721:string, "MFC Mass Flow"=w720:string, "MFC Set Point"=w719:string)  [unwired: 10 in]
        n158 = call "MFC_Data_Process.vi"("MFC"=w724) -> ("MFC Absolute Pressure"=w718:string, "MFC Temperature"=w717:string, "MFC Volumetric Flow"=w716:string, "MFC Mass Flow"=w715:string, "MFC Set Point"=w714:string)  [unwired: 10 in]
        n159 = local read "Flight Number"() -> (w677:string)
        n160 = To Unsigned Long Integer(number=w746) -> (unsigned 32bit integer=w740:u32)
        n161 = To Unsigned Long Integer(number=w745) -> (unsigned 32bit integer=w739:u32)
        n162 = Number To Fractional String(number=w751, precision (6)=i16 5) -> (F-format string=w748:string)  [unwired: 2 in]
        n163 = Number To Fractional String(number=w749, precision (6)=i16 5) -> (F-format string=w747:string)  [unwired: 2 in]
        n164 = local read "MFC_3 SLPM set value"() -> (w680:dbl)
        n165 = Number To Decimal String(number=w740) -> (decimal integer string=w743:string)  [unwired: 1 in]
        n166 = Number To Decimal String(number=w739) -> (decimal integer string=w741:string)  [unwired: 1 in]
        n167 = Replace Array Subset(array=w738, new element=w801, index=w737) -> (w731:string[])
        "Data Array TCP" <- w731
        n168 = Concatenate Strings(w778, w787, "\r") -> ()  [unwired: 1 out]
        n169 = Number To Fractional String(number=w682, precision (6)=i16 2) -> (F-format string=w681:string)  [unwired: 2 in]
        n170 = case shown="True" "Clear Display\nErrors" {
          frame False {
          }
          frame True {
            w859 = errorcluster {"status"=FALSE, "code"=0, "source"=""} ("UDP Error Out")
            n171 = local write "SEPTIC TCP Error Out"(w859) -> ()
            n172 = local write "Serial Visa Error"(w859) -> ()
            n173 = local write "FISH TCP Error Out"(w859) -> ()
            n174 = local write "UDP_Out_Error"(w859) -> ()
          }
        }
        n175 = Index Array(array=w731, index=0) -> (element=w735:string)
        n176 = Scan From String(format string="%f", input string=w735) -> (error out=w727:errorcluster, output 1=w733:dbl)  [unwired: 3 in, 2 out]
        n177 = Unbundle(w727) -> ("status"=w726:bool)  [unwired: 2 out]
        n178 = case shown="False" w726 {
          tunnel: w733 -> [w847 _]
          tunnel: [w846 ""] -> w732
          tunnel: [w845 0.0 ("Output")] -> w728
          frame False {
            n179 = local read "Offset"() -> (w843:dbl)
            n180 = local read "Slope"() -> (w844:dbl)
            n181 = call "SO2 Calibration Equation.vi"("Input"=w847, "Offset"=w843, "Slope"=w844) -> ("Output"=w845:dbl)  [unwired: 12 in]
            n182 = Number To Fractional String(number=w845, precision (6)=i16 5) -> (F-format string=w846:string)  [unwired: 2 in]
          }
          frame True {
          }
        }
        n183 = case shown="True" w757 {
          tunnel: w756 -> [_ w858]
          tunnel: w728 -> [_ w855]
          tunnel: w728 -> [_ w857]
          tunnel: w755 -> [_ w856]
          frame False {
          }
          frame True {
            # "SO2 monitor every second"
            n184 = Lossy Enqueue Element(queue=w858, element=w855) -> ()  [unwired: 1 in, 4 out]
            n185 = Lossy Enqueue Element(queue=w856, element=w857) -> ()  [unwired: 1 in, 4 out]
          }
        }
        n186 = Number To Fractional String(number=w680, precision (6)=i16 2) -> (F-format string=w679:string)  [unwired: 2 in]
        n187 = local read "Stop File Write"() -> (w699:bool)
        n188 = call "SO2 TCP Packet_v2.vi"("ID"=w786, "Version"=w785, "utc_time"=w767, "dummy1"="dummy1", "dummy2"="dummy2", "Flight Number"=w677, "Data Array"=w731) -> ("TCP Binary Packet"=w769:string)  [unwired: 8 in]
        "TCP Binary Packet" <- w769
        n189 = Replace Array Subset(array=w731, new element=w732, index=0) -> (w730:string[])
        "Data Array UDP" <- w730
        n190 = Array To Spreadsheet String(delimiter (Tab)=",", array=w730, 3:"%s" ("format string")) -> (spreadsheet string=w797:string)
        n191 = Enqueue Element(queue=w771, element=w769, error in (no error)=w770) -> ()  [unwired: 1 in, 3 out]
        n192 = Enqueue Element(queue=w783, element=w769, error in (no error)=w782) -> ()  [unwired: 1 in, 3 out]
        n193 = local read "stop"() -> (w810:bool)
        n194 = call <vilib>:"Trim Whitespace.vi"("string"=w797, "location (both)"=w798) -> ("trimmed string"=w760:string)
        "Data String" <- w760
        n195 = Concatenate Strings(w766, w668, w678, w668, w694, w668, w677, w668, w670, w668, w669, w668, w760, w668, w748, w668, w747, w668, w743, w668, w741, w668, w723, w668, w722, w668, w721, w668, w720, w668, w719, w668, w718, w668, w717, w668, w716, w668, w715, w668, w714, w668, w674, w668, w681, w668, w679) -> (w803:string)
        n196 = String Length(string=w803) -> (length=w807:i32)
        n197 = Number To Decimal String(number=w807, width (-)=i16 3) -> (decimal integer string=w805:string)
        n198 = Concatenate Strings(w786, w785, w804, w805, w804, w803) -> (w700:string)
        "UDP_ASCII_Out" <- w700
        n199 = case shown="False" w699 {
          tunnel: w700 -> [w838 _]
          tunnel: w707 -> [w840 w842]
          tunnel: w706 -> [w839 w841]
          tunnel: [w835 _] -> w702
          tunnel: [w834 _] -> w701
          frame False {
            n200 = Concatenate Strings(w838, "\r") -> (w836:string)
            n201 = Write to Text File(file (use dialog)=w840, text=w836, error in=w839) -> (refnum out=w835:refnum<file>, error out=w834:errorcluster)  [unwired: 2 out]
          }
          frame True {
            n202 = Close File(refnum=w842, error in=w841) -> ()  [unwired: 2 out]
          }
        }
        n203 = case shown="True" w757 {
          tunnel: w781 -> [_ w862]
          tunnel: w780 -> [_ w861]
          tunnel: w700 -> [_ w860]
          frame False {
          }
          frame True {
            # "Send UDP data once\na second"
            n204 = Enqueue Element(queue=w862, element=w860, error in (no error)=w861) -> ()  [unwired: 1 in, 3 out]
          }
        }
        n205 = node-c288() -> ()  [unwired: 1 in, 1 out]
      }
      n206 = node-c288() -> (w62:T3)  [unwired: 4 in]
      n207 = node-c288() -> (w64:T3)  [unwired: 4 in]
      n208 = while {
        tunnel: [w527] -> w91
        tunnel: w60 -> [w540]
        tunnel: w59 -> [w539]
        tunnel: [w538] -> w90
        tunnel: w87 -> [w537]
        shift-right: [w535] -> _
        shift-left: 0 -> [w536]
        shift-right: [w533] -> _
        shift-left: u32 0 -> [w534]
        tunnel: w71 -> [w525]
        stop <- "stop" stop-if-true
        w528 = 2
        w530 = string[] ["pmt voltage", "lamp voltage", "lamp int", "internal temp", "react temp", "pres", "flow", "flags"]
        # ">>Monitor command enter as a pair>>"
        # ">>Main commands>>"
        # ">>Monitor Command>>"
        n209 = Array Size(array=w530) -> (size(s)=w531:i32)
        n210 = Divide(x=w531, y=w528) -> (x/y=w529:dbl)
        n211 = for {
          N: w529 -> [_]
          tunnel: w540 -> [w550]
          tunnel: w539 -> [w549]
          tunnel: [w559] -> w527
          shift-right: [w557] -> w535
          shift-left: w536 -> [w558]
          shift-right: [w555] -> w533
          shift-left: w534 -> [w556]
          tunnel: [w554] -> w538
          tunnel: w537 -> [w553]
          tunnel: w530 -> [w546]
          tunnel: "so2" -> [w551]
          tunnel: w528 -> [w547]
          tunnel: w525 -> [w541]
          i -> [w548]
          # "FOR Loop runs according\nto the number of monitor commands"
          # "Assemble command:\nso2\npmt voltage\nlamp voltage\n\netc\netc\n\nso2\nflow\nflags"
          n212 = Multiply(x=w547, y=w548) -> (x*y=w544:i32)
          n213 = Array Subset(array=w546, index=w544, length=w547) -> (w545:string[])
          n214 = Build Array (concatenate)(w551, w545) -> (w552:string[])
          "Data In Array" <- w552
          n215 = node-c288() -> (w543:T3)  [unwired: 4 in]
          n216 = timed-sequence {
            timing: w543 -> [_]
            timing-out: [_] -> w542
            tunnel: w558 -> [w581]
            tunnel: w552 -> [w580]
            tunnel: w550 -> [w579]
            tunnel: w549 -> [w578]
            tunnel: w544 -> [w577]
            tunnel: w553 -> [w572]
            tunnel: [w568] -> w559
            tunnel: [w566] -> w557
            tunnel: w556 -> [w564]
            tunnel: [w563] -> w555
            tunnel: [w562] -> w554
            tunnel: w541 -> [w560]
            n217 = timed-flat-sequence {
              tunnel: w580 -> [w586]
              tunnel: w581 -> [w587]
              tunnel: [w584] -> w576
              tunnel: [w587] -> w575
              tunnel: [w586] -> w574
              tunnel: [w585] -> w573
              tunnel: w579 -> [w584]
              tunnel: [w583] -> w571
              tunnel: w578 -> [w583]
              tunnel: [w582] -> w570
              tunnel: w577 -> [w582]
              tunnel: [w600] -> w569
              tunnel: [w597] -> w567
              tunnel: w576 -> [w592]
              tunnel: w575 -> [w599]
              tunnel: w574 -> [w598]
              tunnel: [w596] -> w565
              tunnel: w573 -> [w596]
              tunnel: [w595] -> w561
              tunnel: w572 -> [w594]
              tunnel: w571 -> [w593]
              tunnel: w570 -> [w591]
              tunnel: w560 -> [w590]
              tunnel: [w662] -> w566
              tunnel: [w663] -> w568
              tunnel: w569 -> [w663]
              tunnel: w567 -> [w662]
              tunnel: w565 -> [w658]
              tunnel: w564 -> [w657]
              tunnel: [w656] -> w563
              tunnel: [w655] -> w562
              tunnel: w561 -> [w655]
              frame #0 {
                n218 = node-c288() -> ()  [unwired: 1 in, 1 out]
                n219 = node-c288() -> ()  [unwired: 1 in, 1 out]
                n220 = Tick Count (ms)() -> (millisecond timer value=w585:u32)
              }
              frame #1 {
                n221 = node-c288() -> ()  [unwired: 1 in, 1 out]
                n222 = while {
                  tunnel: [w614] -> w600
                  tunnel: w598 -> [w612]
                  tunnel: [w610] -> w595
                  tunnel: w594 -> [w609]
                  tunnel: w593 -> [w608]
                  tunnel: w592 -> [w607]
                  tunnel: w591 -> [w606]
                  shift-right: [w611] -> w597
                  shift-left: w599 -> [w613]
                  tunnel: w590 -> [w603]
                  stop <- TRUE stop-if-true
                  # "Receive data is organised as:\nDate Time so2 DATA -1\nDate Time pmt voltage DATA 0\nDate Time lamp voltage DATA 1\nDate Time so2 DATA -1\nDate Time lamp int DATA 2\nDate Time internal temp DATA 3\nDate Time so2 DATA -1\nDate Time react temp DATA 4\nDate Time pres DATA 5\nDate Time so2 DATA -1\nDate Time flow DATA 6\nDate Time flags DATA 7\n\nDate Time Read Error -2"
                  n223 = for {
                    tunnel: w608 -> [w631]
                    tunnel: [w632] -> w614
                    tunnel: w612 -> [w629] mode=indexing
                    tunnel: [w633] -> w610
                    tunnel: w609 -> [w639]
                    tunnel: w607 -> [w634]
                    tunnel: w606 -> [w628]
                    shift-right: [w643] -> w611
                    shift-left: w613 -> [w644]
                    tunnel: w603 -> [w617]
                    i -> [w621]
                    # "Acquire every 330msec for 3 times\nto make 1 second"
                    # "SO2 Acquisition Loop"
                    n224 = call "Wait"("Count(mSec)"=w617) -> ()  [unwired: 1 out]
                    n225 = Concatenate Strings("ID", w629, "\r") -> (w627:string)
                    "Command In" <- w627
                    n226 = call "SO2 Serial Packet Write.vi"("VISA resource name In"=w634, "Data in"=w627, "error in (no error)"=w631) -> ("VISA resource name Out"=w636:refnum<visa-resource-name>, "error out"=w635:errorcluster)  [unwired: 11 in]
                    n227 = call "SO2 Serial Packet Read.vi"("VISA resource In"=w636, "error in"=w635) -> ("VISA resource Out"=w633:refnum<visa-resource-name>, "Data Out"=w624:string, "error out"=w632:errorcluster)  [unwired: 11 in]
                    "RAW DATA" <- w624
                    n228 = Equal?(x=w624, y="Read Error") -> (x = y?=w622:bool)
                    n229 = Get Date/Time In Seconds() -> (seconds since 1Jan1904=w616:timestamp)
                    n230 = case shown="False" w622 {
                      tunnel: [w647 "-2"] -> w637
                      tunnel: w621 -> [w646 _]
                      tunnel: w628 -> [w645 _]
                      frame False {
                        n231 = case shown="0" w646 {
                          tunnel: ["-1" w651 w653] -> w647
                          tunnel: w645 -> [_ w649 w652]
                          frame 0 {
                            # "Make internal flag\n-1 represent so2 data"
                          }
                          frame 2 {
                            # "Make internal flag"
                            n232 = Increment(x=w649) -> (x+1=w650:i32)
                            n233 = Number To Decimal String(number=w650) -> (decimal integer string=w651:string)  [unwired: 1 in]
                          }
                          frame 1, Default {
                            # "Make internal flag"
                            n234 = Number To Decimal String(number=w652) -> (decimal integer string=w653:string)  [unwired: 1 in]
                          }
                        }
                      }
                      frame True {
                      }
                    }
                    n235 = Increment(x=w644) -> (x+1=w640:i32)
                    n236 = Unbundle(w632) -> ("status"=w641:bool)  [unwired: 2 out]
                    n237 = call <vilib>:"Trim Whitespace.vi"("string"=w624) -> ("trimmed string"=w638:string)  [unwired: 1 in]
                    n238 = To Unsigned Long Integer(number=w616) -> (unsigned 32bit integer=w620:u32)
                    n239 = Subtract(x=w620, y=u32 2082844800) -> (x-y=w615:u32)
                    n240 = Select(t=w640, s=w641, f=w644) -> (s? t:f=w643:i32)
                    n241 = call <vilib>:"Space Constant.vi"() -> ("String"=w625:string)
                    n242 = Number To Decimal String(number=w615) -> (decimal integer string=w618:string)  [unwired: 1 in]
                    n243 = Build Array(w618, w625, w638, w625, w637) -> (w626:string[])
                    n244 = Enqueue Element(queue=w639, element=w626) -> ()  [unwired: 2 in, 3 out]
                  }
                  "Number of Send & Read Error\nfrom Acquire Loop" <- w611
                  n245 = call "Wait Until Next Multiple"("Count(mSec)"=u32 1000) -> ()  [unwired: 1 out]
                }
                n246 = node-c288() -> ()  [unwired: 1 in, 1 out]
              }
              frame #2 {
                n247 = node-c288() -> ()  [unwired: 1 in, 1 out]
                n248 = Tick Count (ms)() -> (millisecond timer value=w661:u32)
                n249 = Subtract(x=w661, y=w658) -> (x-y=w660:u32)
                "Acq Time" <- w660
                "Time taken history" <- w660
                n250 = Greater?(x=w660, y=w657) -> (0:w659:bool)
                n251 = Select(t=w660, s=w659, f=w657) -> (s? t:f=w656:u32)
                "Max Acq Time diff" <- w656
                n252 = node-c288() -> ()  [unwired: 1 in, 1 out]
              }
            }
          }
          n253 = node-c288(w542) -> ()  [unwired: 1 out]
        }
      }
      n254 = timed-loop {
        tunnel: w68 -> [w352]
        timing: w62 -> [_]
        timing-out: [_] -> w61
        stop <- w353 stop-if-true
        # "10 minutes SO2 Average calculated every second"
        n255 = node-c288() -> ()  [unwired: 1 in, 1 out]
        n256 = Get Queue Status(queue=w352, return elements? (F)=TRUE) -> (elements=w343:dbl[])  [unwired: 1 in, 7 out]
        n257 = for {
          tunnel: w343 -> [w356] mode=indexing
          tunnel: [w360] -> w349
          shift-right: [w359] -> w347
          shift-left: i64 0 -> [w358]
          i -> [w360]
          n258 = To Quad Integer(1:w356) -> (0:w357:i64)
          n259 = Add(x=w358, y=w357) -> (x+y=w359:i64)
        }
        n260 = Increment(x=w349) -> (x+1=w344:i32)
        "q_size" <- w344
        n261 = To Double Precision Float(number=w347) -> (double precision float=w345:dbl)
        n262 = To Double Precision Float(number=w344) -> (double precision float=w346:dbl)
        n263 = Divide(x=w345, y=w346) -> (x/y=→"10min_so2_avg":dbl)
        n264 = local read "stop"() -> (w353:bool)
        n265 = node-c288() -> ()  [unwired: 1 in, 1 out]
      }
      n266 = timed-loop {
        tunnel: w67 -> [w372]
        timing: w64 -> [_]
        timing-out: [_] -> w63
        stop <- w373 stop-if-true
        # "8 hours SO2 Average calculated every second"
        n267 = node-c288() -> ()  [unwired: 1 in, 1 out]
        n268 = Get Queue Status(queue=w372, return elements? (F)=TRUE) -> (elements=w369:dbl[])  [unwired: 1 in, 7 out]
        n269 = for {
          tunnel: w369 -> [w376] mode=indexing
          tunnel: [w380] -> w368
          shift-right: [w379] -> w366
          shift-left: i64 0 -> [w378]
          i -> [w380]
          n270 = To Quad Integer(1:w376) -> (0:w377:i64)
          n271 = Add(x=w378, y=w377) -> (x+y=w379:i64)
        }
        n272 = Increment(x=w368) -> (x+1=w363:i32)
        "q_size 2" <- w363
        n273 = To Double Precision Float(number=w366) -> (double precision float=w364:dbl)
        n274 = To Double Precision Float(number=w363) -> (double precision float=w365:dbl)
        n275 = Divide(x=w364, y=w365) -> (x/y=→"8hr_so2_avg 2":dbl)
        n276 = local read "stop"() -> (w373:bool)
        n277 = node-c288() -> ()  [unwired: 1 in, 1 out]
      }
      n278 = node-c288(w63) -> ()  [unwired: 1 out]
      n279 = node-c288(w61) -> ()  [unwired: 1 out]
      n280 = while {
        stop <- FALSE stop-if-true
        # "CAL MFC 3 status & control"
        n281 = Wait (ms)(milliseconds to wait=u32 1000) -> ()  [unwired: 1 out]
        n282 = call-poly "VISA Configure Serial Port"("VISA resource name"="VISA resource name 2", "timeout (10sec)"="timeout (10sec) 2", "termination char\n(0xA = '\\n' = LF)"=u8 13 ("termination char\n(0xA = '\\n' = LF)"), "Enable Termination\nChar (T)"=TRUE ("Enable Termination\nChar (T)"), "baud rate (9600)"=u32 19200) -> ("VISA resource name out"=w284:refnum<visa-resource-name>, "error out"=w280:errorcluster)  [unwired: 9 in]
        n283 = case shown="No Error" w280 {
          selector: w280 -> [w291 w341]
          tunnel: w284 -> [w292 w342]
          tunnel: [w290 w342] -> w283
          tunnel: [w289 w341] -> w282
          frame No Error {
            n284 = node-c288() -> (w287:T3)  [unwired: 4 in]
            n285 = timed-loop {
              tunnel: w292 -> [w315]
              tunnel: w291 -> [w313]
              tunnel: [w306] -> w290
              tunnel: [w301] -> w289
              shift-right: [w302] -> _
              shift-left: FALSE -> [w305]
              timing: w287 -> [_]
              timing-out: [_] -> w286
              shift-right: [w293] -> _
              shift-left: 0.0 -> [w295]
              stop <- w301 stop-if-true
              n286 = node-c288() -> ()  [unwired: 1 in, 1 out]
              n287 = local read "MFC_3 SLPM set value"() -> (w293:dbl)
              n288 = Not Equal?(x=w293, y=w295) -> (x != y?=w294:bool)
              n289 = case shown="True" w294 {
                tunnel: w315 -> [w323 w338]
                tunnel: [w323 w338] -> w314
                tunnel: w313 -> [w322 w337]
                tunnel: [w322 w337] -> w312
                tunnel: "A" -> [w326 w330]
                tunnel: [w324 w327] -> w310
                frame False {
                  n290 = Concatenate Strings(w326, "\r") -> (w324:string)
                }
                frame True {
                  n291 = Multiply(x="MFC_3 SLPM set value", y=u32 64000) -> (x*y=w334:dbl)
                  n292 = Divide(x=w334, y=u32 5) -> (x/y=w332:dbl)
                  n293 = To Unsigned Long Integer(number=w332) -> (unsigned 32bit integer=w331:u32)
                  n294 = Number To Decimal String(number=w331) -> (decimal integer string=w329:string)  [unwired: 1 in]
                  n295 = Concatenate Strings(w330, w329, "\r") -> (w327:string)
                }
              }
              n296 = VISA Flush I/O Buffer(VISA resource name=w314, error in (no error)=w312) -> (VISA resource name out=w317:refnum<visa-resource-name>, error out=w316:errorcluster)  [unwired: 1 in]
              n297 = Select(t=FALSE, s=w305, f=TRUE) -> (s? t:f=w302:bool)
              "status" <- w302
              n298 = VISA Write(VISA resource name=w317, write buffer=w310, error in (no error)=w316) -> (VISA resource name out=w309:refnum<visa-resource-name>, error out=w308:errorcluster)  [unwired: 1 out]
              n299 = VISA Flush I/O Buffer(VISA resource name=w309, error in (no error)=w308) -> (VISA resource name out=w319:refnum<visa-resource-name>, error out=w318:errorcluster)  [unwired: 1 in]
              n300 = VISA Read(VISA resource name=w319, byte count=u32 50, error in (no error)=w318) -> (VISA resource name out=w306:refnum<visa-resource-name>, read buffer=w300:string, error out=w301:errorcluster)  [unwired: 1 out]
              "Value Read 3" <- w300
              n301 = call <vilib>:"Space Constant.vi"() -> ("String"=w299:string)
              n302 = Spreadsheet String To Array(delimiter (Tab)=w299, format string="%f", spreadsheet string=w300, array type (2D Dbl)=dbl[] []) -> (array=→"MFC 3":dbl[])
              n303 = node-c288() -> ()  [unwired: 1 in, 1 out]
            }
            n304 = node-c288(w286) -> ()  [unwired: 1 out]
          }
          frame Error {
          }
        }
        n305 = VISA Close(VISA resource name=w283, error in (no error)=w282) -> (error out=→"error out 3":errorcluster)
      }
      n306 = while {
        stop <- FALSE stop-if-true
        # "CAL MFC 2 status & control"
        n307 = Wait (ms)(milliseconds to wait=u32 1000) -> ()  [unwired: 1 out]
        n308 = call-poly "VISA Configure Serial Port"("VISA resource name"="VISA resource name 3", "timeout (10sec)"="timeout (10sec) 3", "termination char\n(0xA = '\\n' = LF)"=u8 13 ("termination char\n(0xA = '\\n' = LF)"), "Enable Termination\nChar (T)"=TRUE ("Enable Termination\nChar (T)"), "baud rate (9600)"=u32 19200) -> ("VISA resource name out"=w214:refnum<visa-resource-name>, "error out"=w210:errorcluster)  [unwired: 9 in]
        n309 = case shown="No Error" w210 {
          selector: w210 -> [w221 w271]
          tunnel: w214 -> [w222 w272]
          tunnel: [w220 w272] -> w213
          tunnel: [w219 w271] -> w212
          frame No Error {
            n310 = node-c288() -> (w217:T3)  [unwired: 4 in]
            n311 = timed-loop {
              tunnel: w222 -> [w245]
              tunnel: w221 -> [w243]
              tunnel: [w236] -> w220
              tunnel: [w231] -> w219
              shift-right: [w232] -> _
              shift-left: FALSE -> [w235]
              timing: w217 -> [_]
              timing-out: [_] -> w216
              shift-right: [w223] -> _
              shift-left: 0.0 -> [w225]
              stop <- w231 stop-if-true
              n312 = node-c288() -> ()  [unwired: 1 in, 1 out]
              n313 = local read "MFC_2 SLPM set value"() -> (w223:dbl)
              n314 = Not Equal?(x=w223, y=w225) -> (x != y?=w224:bool)
              n315 = case shown="True" w224 {
                tunnel: w245 -> [w253 w268]
                tunnel: [w253 w268] -> w244
                tunnel: w243 -> [w252 w267]
                tunnel: [w252 w267] -> w242
                tunnel: "A" -> [w256 w260]
                tunnel: [w254 w257] -> w240
                frame False {
                  n316 = Concatenate Strings(w256, "\r") -> (w254:string)
                }
                frame True {
                  n317 = Multiply(x="MFC_2 SLPM set value", y=u32 64000) -> (x*y=w264:dbl)
                  n318 = Divide(x=w264, y=u32 5) -> (x/y=w262:dbl)
                  n319 = To Unsigned Long Integer(number=w262) -> (unsigned 32bit integer=w261:u32)
                  n320 = Number To Decimal String(number=w261) -> (decimal integer string=w259:string)  [unwired: 1 in]
                  n321 = Concatenate Strings(w260, w259, "\r") -> (w257:string)
                }
              }
              n322 = Select(t=FALSE, s=w235, f=TRUE) -> (s? t:f=w232:bool)
              "status 2" <- w232
              n323 = VISA Flush I/O Buffer(VISA resource name=w244, error in (no error)=w242) -> (VISA resource name out=w247:refnum<visa-resource-name>, error out=w246:errorcluster)  [unwired: 1 in]
              n324 = VISA Write(VISA resource name=w247, write buffer=w240, error in (no error)=w246) -> (VISA resource name out=w239:refnum<visa-resource-name>, error out=w238:errorcluster)  [unwired: 1 out]
              n325 = VISA Flush I/O Buffer(VISA resource name=w239, error in (no error)=w238) -> (VISA resource name out=w249:refnum<visa-resource-name>, error out=w248:errorcluster)  [unwired: 1 in]
              n326 = VISA Read(VISA resource name=w249, byte count=u32 50, error in (no error)=w248) -> (VISA resource name out=w236:refnum<visa-resource-name>, read buffer=w230:string, error out=w231:errorcluster)  [unwired: 1 out]
              "Value Read 2" <- w230
              n327 = call <vilib>:"Space Constant.vi"() -> ("String"=w229:string)
              n328 = Spreadsheet String To Array(delimiter (Tab)=w229, format string="%f", spreadsheet string=w230, array type (2D Dbl)=dbl[] []) -> (array=→"MFC 2":dbl[])
              n329 = node-c288() -> ()  [unwired: 1 in, 1 out]
            }
            n330 = node-c288(w216) -> ()  [unwired: 1 out]
          }
          frame Error {
          }
        }
        n331 = VISA Close(VISA resource name=w213, error in (no error)=w212) -> (error out=→"error out 2":errorcluster)
      }
      n332 = node-c288(w88) -> ()  [unwired: 1 out]
      n333 = while {
        stop <- FALSE stop-if-true
        n334 = node-c288() -> (w93:T3)  [unwired: 4 in]
        n335 = Create Network Stream Reader Endpoint(7:10 ("reader buffer size"), 9:T2 {"Message"="", "Message Data"=variant} ("Message Cluster"), 11:"/command/reader/SO2" ("reader url")) -> (0:w99:errorcluster, 3:w100:refnum<k21>)  [unwired: 4 in]
        n336 = timed-loop "Host->Target Command Reader" {
          shift-right: [w110] -> w97
          shift-left: w99 -> [w113]
          shift-right: [w111] -> w96
          shift-left: w100 -> [w112]
          tunnel: [TRUE] -> _
          timing: w93 -> [_]
          timing-out: [_] -> w92
          stop <- w104 stop-if-true
          # "Receive Commands from Host VI"
          n337 = node-c288() -> ()  [unwired: 1 in, 1 out]
          n338 = shared-variable-read(w112, w113) -> (w111:refnum<k21>, w106:errorcluster, w108:bool, w109:T2)  [unwired: 1 in]
          n339 = Or(x=w108, y=w106) -> (x .or. y?=w107:bool)
          n340 = case shown="False" w107 {
            selector: w107 -> [_ w199]
            tunnel: w106 -> [w121 w200]
            tunnel: [w120 w200] -> w110
            tunnel: w109 -> [w118 _]
            tunnel: [w119 w199] -> w104
            frame False {
              n341 = Unbundle By Name(w118) -> ("Message"=w117:string, "Message Data"=w116:variant)
              n342 = case shown="\"UDP Time Offset\"" w117 {
                tunnel: w121 -> [w123 w128 w133 w138 w143 w148 w153 w158 w163 w168 w173 w178 w183 w188 w193 w197]
                tunnel: [w123 w127 w132 w137 w142 w147 w152 w157 w162 w167 w172 w177 w182 w187 w192 w195] -> w120
                tunnel: w116 -> [_ w126 w131 w136 w141 w146 w151 w156 w161 w166 w171 w176 w181 w186 w191 w198]
                tunnel: [TRUE _ _ _ _ _ _ _ _ _ _ _ _ _ _ _] -> w119
                frame "Stop", Default {
                }
                frame "V9" {
                  n343 = Variant To Data(error in=w128, type=FALSE, Variant=w126) -> (data=w124:bool, error out=w127:errorcluster)
                  "V9" <- w124
                  n344 = shared-variable "NI-cRIO9022-019C2C95\\Mod6\\DO7"(w124) -> ()  [unwired: 1 in, 1 out]
                }
                frame "MFC_2" {
                  n345 = Variant To Data(error in=w133, type=0.0, Variant=w131) -> (data=w129:dbl, error out=w132:errorcluster)
                  n346 = local write "MFC_2 SLPM set value"(w129) -> ()
                }
                frame "MFC_3" {
                  n347 = Variant To Data(error in=w138, type=0.0, Variant=w136) -> (data=w134:dbl, error out=w137:errorcluster)
                  n348 = local write "MFC_3 SLPM set value"(w134) -> ()
                }
                frame "Simulate STEL Conc" {
                  n349 = Variant To Data(error in=w143, type=0.0, Variant=w141) -> (data=→"Simulate STEL Conc":dbl, error out=w142:errorcluster)
                }
                frame "Simulate TWA Conc" {
                  n350 = Variant To Data(error in=w148, type=0.0, Variant=w146) -> (data=→"Simulate TWA Conc":dbl, error out=w147:errorcluster)
                }
                frame "Offset" {
                  n351 = Variant To Data(error in=w153, type=0.0, Variant=w151) -> (data=→"Offset":dbl, error out=w152:errorcluster)
                }
                frame "10mins STEL Limit" {
                  n352 = Variant To Data(error in=w158, type=0, Variant=w156) -> (data=→"10mins_STEL_limit":i32, error out=w157:errorcluster)
                }
                frame "UDP Time Offset" {
                  n353 = Variant To Data(error in=w163, type=0, Variant=w161) -> (data=→"UDP Time Stamp Offset":i32, error out=w162:errorcluster)
                }
                frame "8hr TWA Limit" {
                  n354 = Variant To Data(error in=w168, type=0, Variant=w166) -> (data=→"8hr_TWA_limit":i32, error out=w167:errorcluster)
                }
                frame "Slope" {
                  n355 = Variant To Data(error in=w173, type=0.0, Variant=w171) -> (data=→"Slope":dbl, error out=w172:errorcluster)
                }
                frame "V8" {
                  n356 = Variant To Data(error in=w178, type=FALSE, Variant=w176) -> (data=w174:bool, error out=w177:errorcluster)
                  "V8" <- w174
                  n357 = shared-variable "NI-cRIO9022-019C2C95\\Mod6\\DO6"(w174) -> ()  [unwired: 1 in, 1 out]
                }
                frame "Stop File Write" {
                  n358 = Variant To Data(error in=w183, type=FALSE, Variant=w181) -> (data=→"Stop File Write":bool, error out=w182:errorcluster)
                }
                frame "Flight Number" {
                  n359 = Variant To Data(error in=w188, type="", Variant=w186) -> (data=→"Flight Number":string, error out=w187:errorcluster)
                }
                frame "V6" {
                  n360 = Variant To Data(error in=w193, type=FALSE, Variant=w191) -> (data=w189:bool, error out=w192:errorcluster)
                  "V6" <- w189
                  n361 = shared-variable "NI-cRIO9022-019C2C95\\Mod6\\DO4"(w189) -> ()  [unwired: 1 in, 1 out]
                }
                frame "Simulate Conc" {
                  n362 = Variant To Data(error in=w197, type=FALSE, Variant=w198) -> (data=→"Simulate\nconc":bool, error out=w195:errorcluster)
                }
              }
            }
            frame True {
            }
          }
          n363 = node-c288() -> ()  [unwired: 1 in, 1 out]
        }
        n364 = node-c288(w92) -> ()  [unwired: 1 out]
        n365 = Destroy Stream Endpoint(8:w97, 11:w96) -> (0:→"error out 4":errorcluster)
        n366 = Wait (ms)(milliseconds to wait=u32 1000) -> ()  [unwired: 1 out]
      }
      n367 = while {
        tunnel: w75 -> [w426]
        stop <- w427 stop-if-true
        # "UDP Broadcast loop"
        # "Broadcast UDP SO2 Data"
        n368 = node-c288() -> (w429:T3)  [unwired: 4 in]
        n369 = String To IP(1:"239.1.4.6" ("name")) -> (0:w431:u32)
        n370 = call-poly <vilib>:"UDP Multicast Open.vi"("time-to-live (1)"=u16 5, "port"=u16 10001) -> ("error out"=w439:errorcluster, "connection ID"=w440:refnum<k16>)  [unwired: 8 in]
        n371 = timed-loop {
          tunnel: w440 -> [w460]
          tunnel: w439 -> [w459]
          tunnel: [w446] -> w435
          shift-right: [w449] -> _
          shift-left: FALSE -> [w452]
          tunnel: [w444] -> w433
          tunnel: w431 -> [w448]
          tunnel: u16 50001 ("port or service name") -> [w447]
          timing: w429 -> [_]
          timing-out: [_] -> w428
          tunnel: [w442] -> w427
          tunnel: w426 -> [w441]
          stop <- w443 stop-if-true
          n372 = node-c288() -> ()  [unwired: 1 in, 1 out]
          n373 = local read "Flight Number"() -> (w455:string)
          n374 = Select(t=FALSE, s=w452, f=TRUE) -> (s? t:f=w449:bool)
          "UDP packet \nstatus" <- w449
          n375 = feedback-in #2(w455) -> ()
          n376 = feedback #2() -> (w454:string)  [unwired: 1 in]
          n377 = Not Equal?(x=w455, y=w454) -> (x != y?=w453:bool)
          n378 = flat-sequence {
            tunnel: w448 -> [w468]
            tunnel: w459 -> [w469]
            tunnel: w460 -> [w470]
            tunnel: [w470] -> w458
            tunnel: [w469] -> w457
            tunnel: [w468] -> w456
            tunnel: w453 -> [w467]
            tunnel: w447 -> [w480]
            tunnel: w458 -> [w479]
            tunnel: w457 -> [w478]
            tunnel: w456 -> [w477]
            tunnel: [w476] -> w446
            tunnel: [w475] -> w444
            tunnel: w441 -> [w474]
            frame #0 {
              n379 = feedback #3(u32 0) -> (w464:u32)
              n380 = case shown="True" w467 {
                tunnel: w464 -> [w471 _]
                tunnel: [w471 u32 0] -> w463
                frame False {
                }
                frame True {
                }
              }
              "UDP_Pack_num" <- w463
              n381 = Increment(x=w463) -> (x+1=w465:u32)
              n382 = feedback-in #3(w465) -> ()
            }
            frame #1 {
              n383 = Dequeue Element(queue=w474) -> (element=w473:string)  [unwired: 2 in, 3 out]
              n384 = UDP Write(address=w477, port or service name=w480, connection ID=w479, data in=w473, 8:w478) -> (error out=w475:errorcluster, 3:w476:refnum<k16>)  [unwired: 1 in]
            }
          }
          n385 = local read "stop"() -> (w442:bool)
          n386 = Unbundle(w444) -> ("status"=w445:bool)  [unwired: 2 out]
          n387 = node-c288() -> ()  [unwired: 1 in, 1 out]
          n388 = Compound Arithmetic op=OR(w445, w442) -> (w443:bool)
        }
        n389 = node-c288(w428) -> ()  [unwired: 1 out]
        n390 = UDP Close(connection ID=w435, 8:w433) -> (error out=→"UDP_Out_Error":errorcluster)  [unwired: 1 out]
        n391 = Wait (ms)(milliseconds to wait=u32 1000) -> ()  [unwired: 1 out]
      }
      n392 = while {
        tunnel: w72 -> [w385]
        tunnel: w73 -> [w384]
        stop <- w388 stop-if-true
        # "TCP Loop writing to SEPTIC Tank"
        n393 = TCP Open Connection(address="192.168.101.108", remote port or service name=u16 3502) -> (connection ID=w391:refnum<k5>, error out=w386:errorcluster)  [unwired: 3 in]
        n394 = case shown="No Error" w386 {
          selector: w386 -> [w396 w423]
          tunnel: w391 -> [w401 w424]
          tunnel: [w400 w424] -> w390
          tunnel: [w399 w423] -> w389
          tunnel: [w398 w422] -> w388
          tunnel: w384 -> [w395 _]
          tunnel: w385 -> [w394 _]
          frame No Error {
            n395 = node-c288() -> (w403:T3)  [unwired: 4 in]
            n396 = timed-loop {
              tunnel: w401 -> [w417]
              tunnel: w396 -> [w416]
              tunnel: [w415] -> w400
              tunnel: [w414] -> w399
              tunnel: [w404] -> w398
              shift-right: [w408] -> _
              shift-left: FALSE -> [w411]
              timing: w403 -> [_]
              timing-out: [_] -> w402
              tunnel: w395 -> [w407]
              tunnel: w394 -> [w406]
              stop <- w412 stop-if-true
              n397 = node-c288() -> ()  [unwired: 1 in, 1 out]
              n398 = Dequeue Element(queue=w407, error in (no error)=w406) -> (element=w405:string)  [unwired: 1 in, 3 out]
              n399 = Select(t=FALSE, s=w411, f=TRUE) -> (s? t:f=w408:bool)
              "TCP packet\nSend to SEPTIC" <- w408
              n400 = TCP Write(connection ID=w417, data in=w405, error in (no error)=w416) -> (connection ID out=w415:refnum<k5>, error out=w414:errorcluster)  [unwired: 1 in, 1 out]
              n401 = local read "stop"() -> (w404:bool)
              n402 = Unbundle(w414) -> ("status"=w413:bool)  [unwired: 2 out]
              n403 = node-c288() -> ()  [unwired: 1 in, 1 out]
              n404 = Compound Arithmetic op=OR(w413, w404) -> (w412:bool)
            }
            n405 = node-c288(w402) -> ()  [unwired: 1 out]
          }
          frame Error {
            n406 = local read "stop"() -> (w422:bool)
          }
        }
        n407 = TCP Close Connection(connection ID=w390, error in (no error)=w389) -> (error out=→"SEPTIC TCP Error Out":errorcluster)  [unwired: 1 in, 1 out]
        n408 = Wait (ms)(milliseconds to wait=u32 1000) -> ()  [unwired: 1 out]
      }
      n409 = while {
        tunnel: w79 -> [w485]
        tunnel: w78 -> [w484]
        stop <- w488 stop-if-true
        # "TCP Loop writing to FISH Tank"
        n410 = TCP Open Connection(address="192.168.101.110", remote port or service name=u16 3502) -> (connection ID=w491:refnum<k5>, error out=w486:errorcluster)  [unwired: 3 in]
        n411 = case shown="No Error" w486 {
          selector: w486 -> [w496 w523]
          tunnel: w491 -> [w501 w524]
          tunnel: [w500 w524] -> w490
          tunnel: [w499 w523] -> w489
          tunnel: [w498 w522] -> w488
          tunnel: w485 -> [w495 _]
          tunnel: w484 -> [w494 _]
          frame No Error {
            n412 = node-c288() -> (w503:T3)  [unwired: 4 in]
            n413 = timed-loop {
              tunnel: w501 -> [w517]
              tunnel: w496 -> [w516]
              tunnel: [w515] -> w500
              tunnel: [w514] -> w499
              tunnel: [w511] -> w498
              shift-right: [w507] -> _
              shift-left: FALSE -> [w510]
              timing: w503 -> [_]
              timing-out: [_] -> w502
              tunnel: w495 -> [w506]
              tunnel: w494 -> [w505]
              stop <- w512 stop-if-true
              n414 = node-c288() -> ()  [unwired: 1 in, 1 out]
              n415 = Dequeue Element(queue=w506, error in (no error)=w505) -> (element=w504:string)  [unwired: 1 in, 3 out]
              n416 = Select(t=FALSE, s=w510, f=TRUE) -> (s? t:f=w507:bool)
              "TCP packet\nSend to FISH" <- w507
              n417 = TCP Write(connection ID=w517, data in=w504, error in (no error)=w516) -> (connection ID out=w515:refnum<k5>, error out=w514:errorcluster)  [unwired: 1 in, 1 out]
              n418 = local read "stop"() -> (w511:bool)
              n419 = Unbundle(w514) -> ("status"=w513:bool)  [unwired: 2 out]
              n420 = node-c288() -> ()  [unwired: 1 in, 1 out]
              n421 = Compound Arithmetic op=OR(w513, w511) -> (w512:bool)
            }
            n422 = node-c288(w502) -> ()  [unwired: 1 out]
          }
          frame Error {
            n423 = local read "stop"() -> (w522:bool)
          }
        }
        n424 = TCP Close Connection(connection ID=w490, error in (no error)=w489) -> (error out=→"FISH TCP Error Out":errorcluster)  [unwired: 1 in, 1 out]
        n425 = Wait (ms)(milliseconds to wait=u32 1000) -> ()  [unwired: 1 out]
      }
    }
    frame Error {
    }
  }
  n426 = VISA Close(VISA resource name=w36, error in (no error)=w35) -> (error out=→"Serial Visa Error":errorcluster)
